vi "From DateTime.vi"(1 "DateTime":timestamp) -> (0 "Formatted DateTime":dbl)   [LabVIEW 2013, in "OPC UA runtime.lvclass"]
doc: "Convert DateTime to data type which can be used by DCAF"
uses:
  OPC UA runtime.lvclass
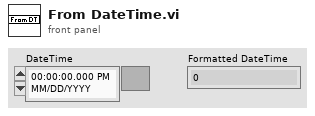
[diagram p1: front panel]
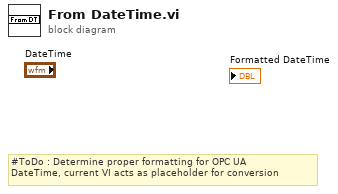
[diagram p0: block diagram]
diagram:
  # "#ToDo : Determine proper formatting for OPC UA\nDateTime, current VI acts as placeholder for conversion"
